vi "VItimingTemplate.vi"() -> ()   [LabVIEW 2021]
panel:
  out "execTime":dbl caption="Execution Time" format="%_3ps"
  # "Open the diagram, Select All, Copy, paste to your VI, put your guts inside the middle frame\n\nCould probably do this automatically if I could be bothered to learn VI scripting!"
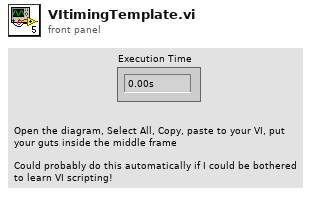
[diagram p1: front panel]
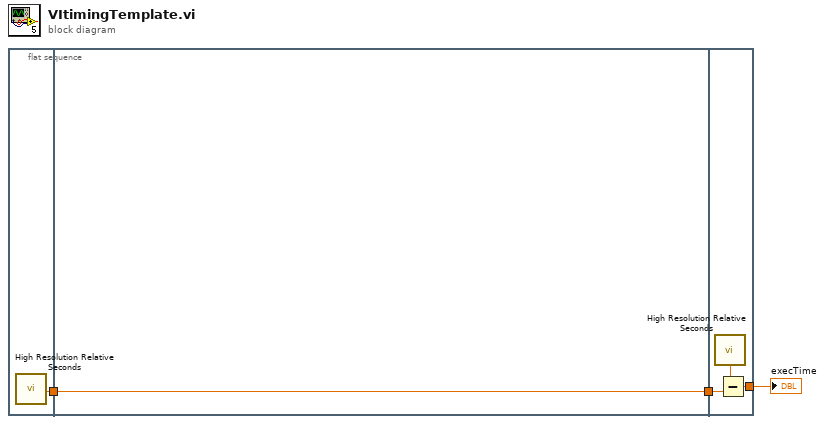
[diagram p0: block diagram]
diagram:
  n1 = flat-sequence {
    tunnel: [w4] -> w3
    tunnel: w3 -> [w5]
    tunnel: [w5] -> w2
    tunnel: w2 -> [w7]
    tunnel: [w6] -> w1
    frame #0 {
      n2 = call <vilib>:"High Resolution Relative Seconds.vi"() -> ("relative seconds"=w4:dbl)
    }
    frame #1 {
    }
    frame #2 {
      n3 = call <vilib>:"High Resolution Relative Seconds.vi"() -> ("relative seconds"=w8:dbl)
      n4 = Subtract(x=w8, y=w7) -> (x-y=w6:dbl)
    }
  }
  "execTime" <- w1
